vi "S2C_FORNAX_Proc_LocalCmd.vi"(8 "Error In":errorcluster, 11 "Q-Ref":refnum<queue>) -> (0 "Error Out":errorcluster, 3 "Command":string)   [LabVIEW 2015]
uses:
  S2C_FORNAX_Proc_Globals.vi
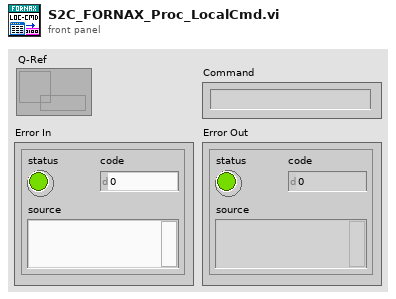
[diagram p1: front panel]
types:
  T1 = cluster{"Caller-Q":refnum<queue>, "Command":string, "Return":string, "Data":variant, "Timeout":dbl}
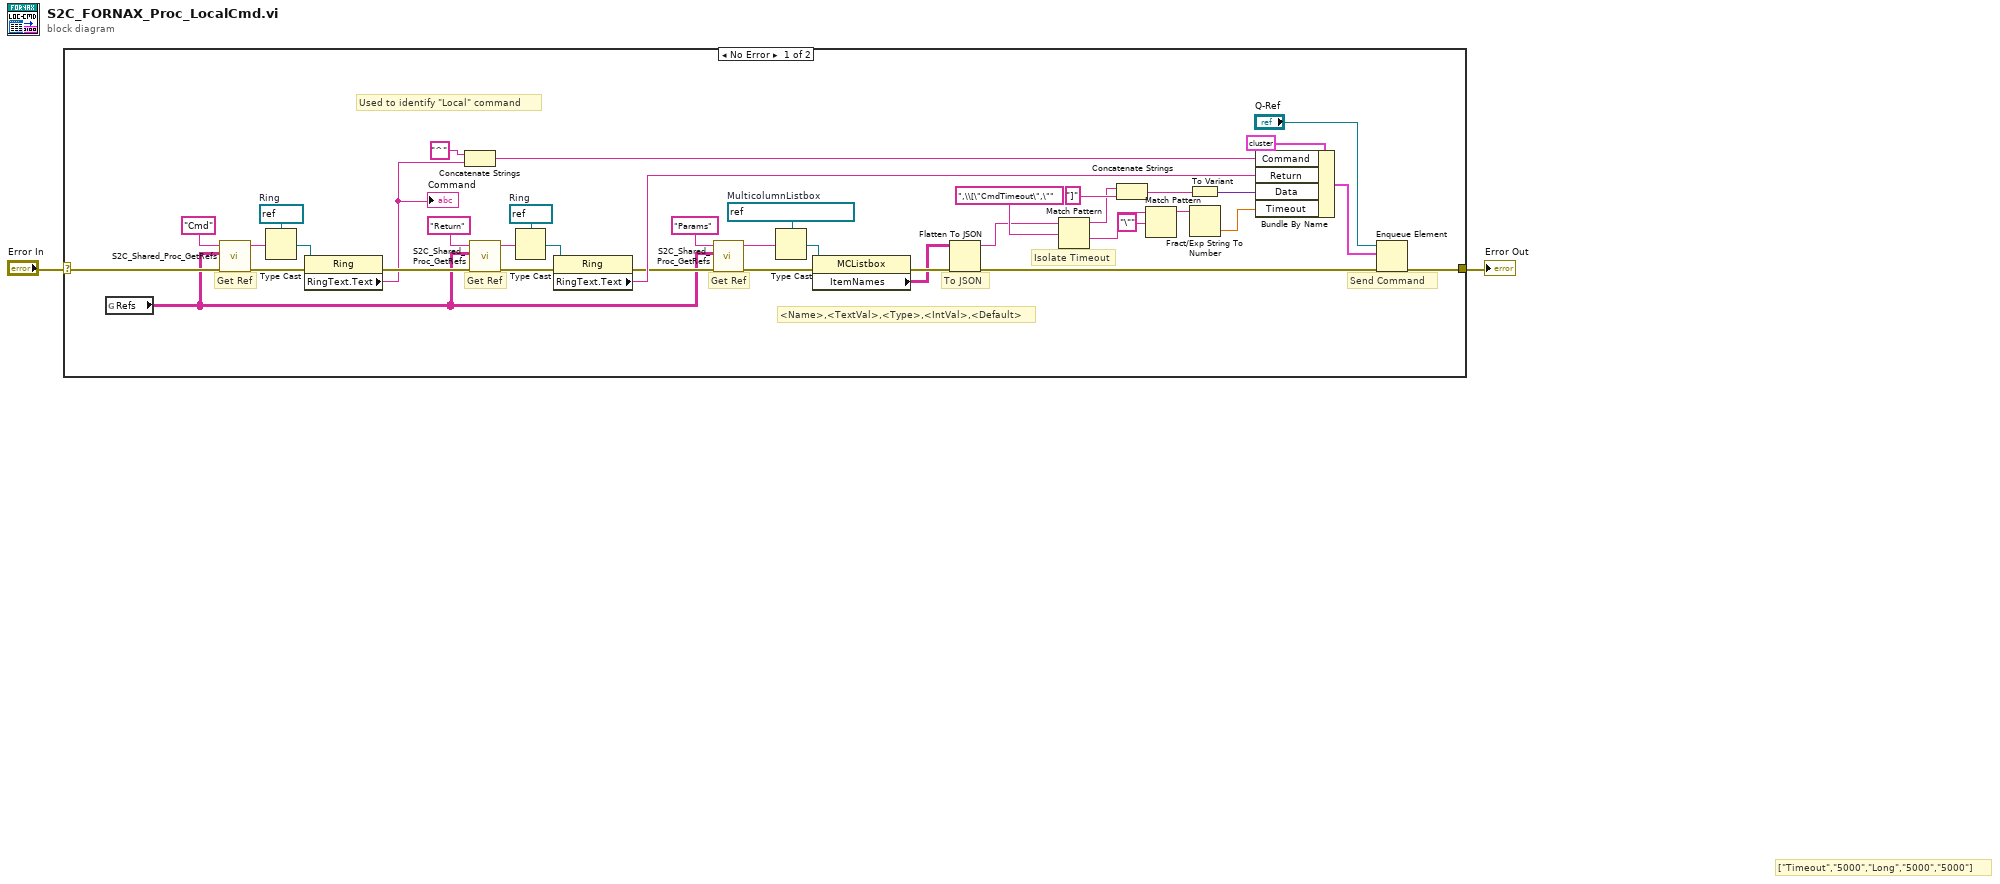
[diagram p0: block diagram]
diagram:
  # "[\"Timeout\",\"5000\",\"Long\",\"5000\",\"5000\"]"
  n1 = case shown="No Error" "Error In" {
    selector: "Error In" -> [w32 w43]
    tunnel: [w40 w43] -> w1
    frame No Error {
      w11 = refnum<vi> refnum  # Ring
      w30 = refnum<vi> refnum  # MulticolumnListbox
      w35 = refnum<vi> refnum  # Ring
      # "Get Ref"
      # "To JSON"
      # "Isolate Timeout"
      # "Get Ref"
      # "Get Ref"
      # "Used to identify \"Local\" command"
      # "<Name>,<TextVal>,<Type>,<IntVal>,<Default>"
      # "Send Command"
      n2 = global read "S2C_FORNAX_Proc_Globals.vi" "Refs"() -> (w4:string[][])
      n3 = call "S2C_Shared_Proc_GetRefs.vi"("Error In"=w32, "Refs"=w4, "Label"="Cmd") -> ("Error Out"=w34:errorcluster, "Reference"=w36:string)  [unwired: 7 in]
      n4 = Type Cast(type=w35, x=w36) -> (*(type *) &x=w37:refnum<vi>)
      n5 = property class="Ring"(reference=w37, error in=w34) -> (error out=w8:errorcluster, "RingText.Text"=w3:string)  [unwired: 1 out]
      "Command" <- w3
      n6 = Concatenate Strings("^" ("string"), w3) -> (w7:string)
      n7 = call "S2C_Shared_Proc_GetRefs.vi"("Error In"=w8, "Refs"=w4, "Label"="Return") -> ("Error Out"=w12:errorcluster, "Reference"=w10:string)  [unwired: 7 in]
      n8 = Type Cast(type=w11, x=w10) -> (*(type *) &x=w9:refnum<vi>)
      n9 = property class="Ring"(reference=w9, error in=w12) -> (error out=w5:errorcluster, "RingText.Text"=w6:string)  [unwired: 1 out]
      n10 = call "S2C_Shared_Proc_GetRefs.vi"("Error In"=w5, "Refs"=w4, "Label"="Params") -> ("Error Out"=w31:errorcluster, "Reference"=w29:string)  [unwired: 7 in]
      n11 = Type Cast(type=w30, x=w29) -> (*(type *) &x=w28:refnum<vi>)
      n12 = property class="MCListbox"(reference=w28, error in=w31) -> (error out=w18:errorcluster, "ItemNames"=w17:string[][])  [unwired: 1 out]
      n13 = Flatten To JSON(anything=w17, error in (no error)=w18) -> (JSON string=w16:string, 11:w14:errorcluster)  [unwired: 1 in]
      n14 = Match Pattern(string=w16, regular expression=",\\[\"CmdTimeout\",\"") -> (before substring=w21:string, after substring=w25:string)  [unwired: 1 in, 2 out]
      n15 = Concatenate Strings(w21, "]" ("string")) -> (w20:string)
      n16 = Match Pattern(string=w25, regular expression="\"") -> (before substring=w23:string)  [unwired: 1 in, 3 out]
      n17 = To Variant(anything=w20) -> (Variant=w19:variant)
      n18 = Fract/Exp String To Number(string=w23) -> (number=w15:dbl)  [unwired: 3 in, 1 out]
      n19 = Bundle By Name(cluster=T1 {"Caller-Q"=refnum, "Command"="", "Return"="None", "Data"=variant, "Timeout"=10.0} ("element"), "Command"=w7, "Return"=w6, "Data"=w19, "Timeout"=w15) -> (w39:T1)
      n20 = Enqueue Element(queue="Q-Ref", element=w39, error in (no error)=w14) -> (error out=w40:errorcluster)  [unwired: 1 in, 2 out]
    }
    frame Error {
    }
  }
  "Error Out" <- w1
